vi "_TEST_Set Excel Values.vi"() -> ()   [LabVIEW 2017, in "excel_configuration.lvlib"]
uses:
  excel_configuration.lvlib
panel:
  in  "data":string[][](array[string])=[["1", "a"], ["2", "b"], ["3", "c"]]
  out "error out":errorcluster
  in  "path":path=path "d:/1234.xlsx"
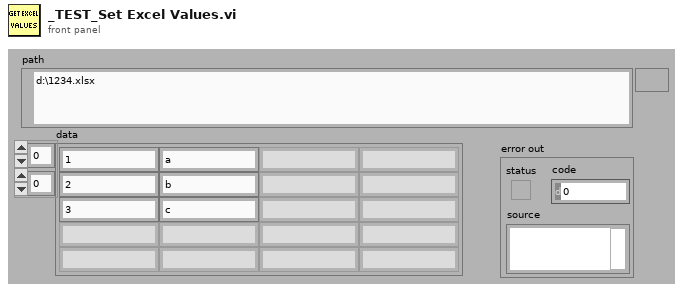
[diagram p1: front panel]
types:
  T1 = cluster{"Excel._Application":refnum<k7>, "Workbooks":refnum<k7>}
  T2 = cluster{"Excel._Application":refnum<k7>, "Workbooks":refnum<k7>, "Open":refnum<k7>}
  T3 = cluster{"Excel._Application":refnum<k7>, "Workbooks":refnum<k7>, "Open":refnum<k7>, "Worksheets":refnum<k7>, "Excel._Worksheet":refnum<k7>}
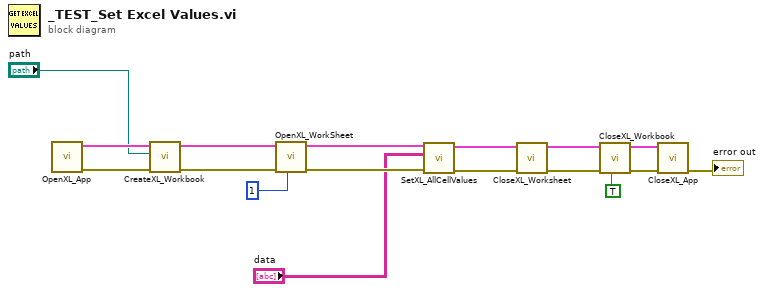
[diagram p0: block diagram]
diagram:
  n1 = call "OpenXL_App.vi"() -> ("error out"=w11:errorcluster, "Refnum Cluster"=w12:T1)  [unwired: 10 in]
  n2 = call "CreateXL_Workbook.vi"("error in"=w11, "path"="path", "Refnum Cluster In"=w12) -> ("error out"=w3:errorcluster, "Refnum Cluster Out"=w4:T2)  [unwired: 7 in]
  n3 = call "OpenXL_WorkSheet.vi"("Sheet"=1, "error in (no error)"=w3, "Refnum Cluster In"=w4) -> ("error out"=w16:errorcluster, "Refnum Cluster Out"=w17:T3)  [unwired: 7 in]
  n4 = call "SetXL_AllCellValues.vi"("error in (no error)"=w16, "data"="data", "Refnum Cluster Out in"=w17) -> ("error out"=w8:errorcluster, "Refnum Cluster Out out"=w9:T3)  [unwired: 7 in]
  n5 = call "CloseXL_Worksheet.vi"("error in (no error)"=w8, "Refnum Cluster In"=w9) -> ("error out"=w6:errorcluster, "Refnum Cluster Out"=w7:T2)  [unwired: 8 in]
  n6 = call "CloseXL_Workbook.vi"("Save? (F)"=TRUE, "error in (no error)"=w6, "Refnum Cluster In"=w7) -> ("error out"=w14:errorcluster, "Refnum Cluster Out"=w15:T1)  [unwired: 7 in]
  n7 = call "CloseXL_App.vi"("error in (no error)"=w14, "Refnum Cluster In"=w15) -> ("error out"=→"error out":errorcluster)  [unwired: 9 in]
